vi "Set 430 Rate.vi"(8 "error in (no error)":errorcluster, 11 "VISA session":refnum<visa-resource-name>="GPIB0::22::INSTR") -> (0 "error out":errorcluster, 3 "VISA session out":refnum<visa-resource-name>="GPIB0::22::INSTR")   [LabVIEW 2021]
panel:
  in  "Slew Rate [T/min]":dbl
  in  "Input Cluster":T1 {"MaxLambdaCurrent [A]" format="%.2f"; "LambdaRates [A/min]" format="%.5e"; "MaxNormalCurrent [A]" format="%.2f"; "StabilitySetting [%]" format="%.2f"; "FieldCurrentRatio [T/A]" format="%.2f"; "SwitchWaitTime [s]" format="%.2f"; "SwitchHtrCurrent [mA]" format="%.2f"; "TrainRates [A/min]" format="%.5e"; "NormalRates [A/min]" format="%.5e"; "Breakpts [A]" format="%.5e"}
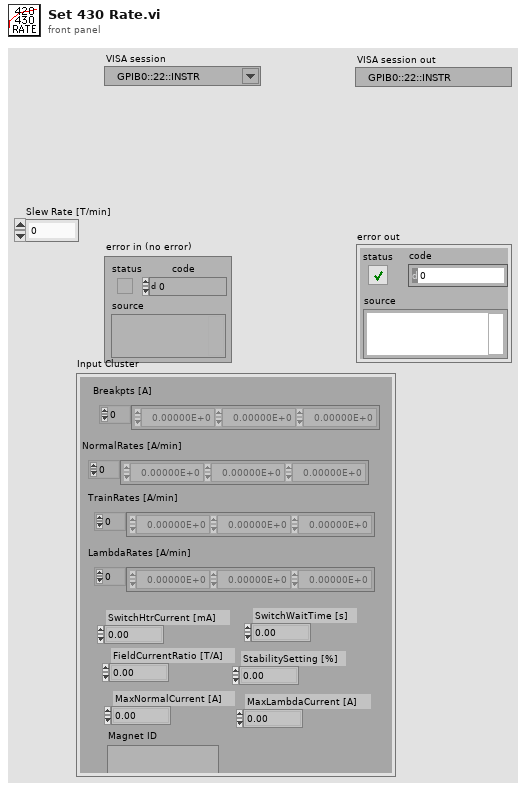
[diagram p1: front panel]
types:
  T1 = cluster{"Breakpts [A]":dbl[], "NormalRates [A/min]":dbl[], "TrainRates [A/min]":dbl[], "SwitchHtrCurrent [mA]":dbl, "SwitchWaitTime [s]":dbl, "FieldCurrentRatio [T/A]":dbl, "StabilitySetting [%]":dbl, "MaxNormalCurrent [A]":dbl, "Magnet ID":string, "LambdaRates [A/min]":dbl[], "MaxLambdaCurrent [A]":dbl}
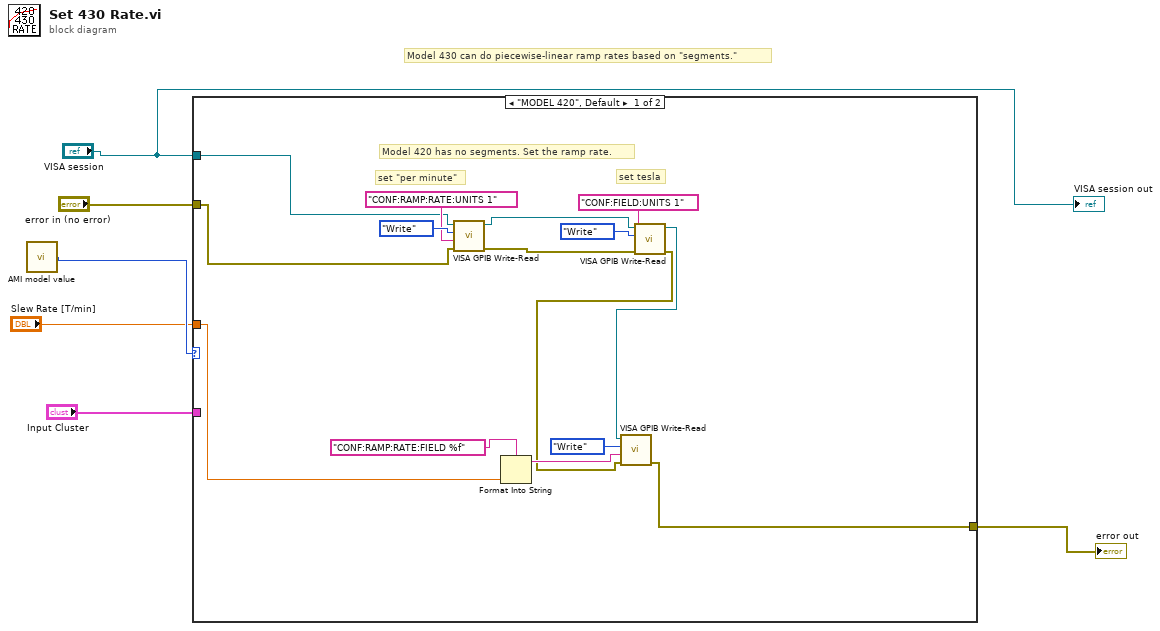
[diagram p0: block diagram]
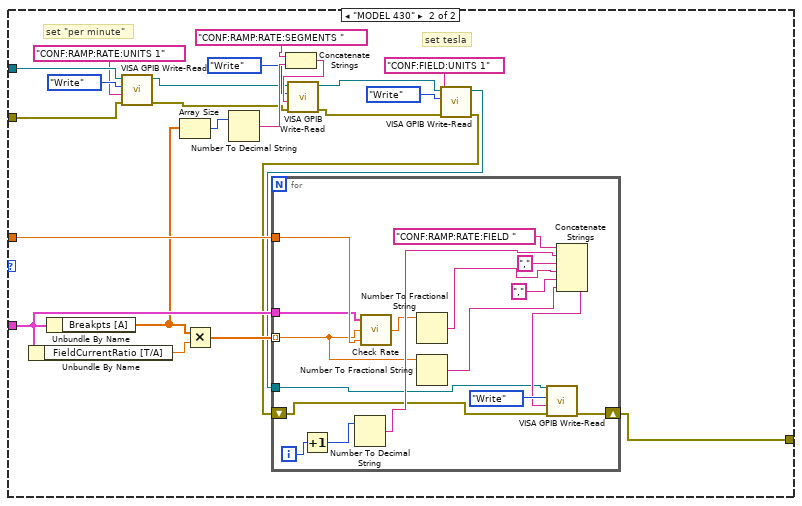
[diagram p2: hidden frame]
diagram:
  # "Model 430 can do piecewise-linear ramp rates based on \"segments.\""
  n1 = call "AMI model value.vi"() -> ("AMI Model 2"=w3:enum16{"MODEL 420", "MODEL 430"})  [unwired: 2 in]
  n2 = case shown="\"MODEL 420\", Default" w3 {
    tunnel: "VISA session" -> [w9 w42]
    tunnel: "error in (no error)" -> [w10 w41]
    tunnel: [w18 w24] -> w5
    tunnel: "Input Cluster" -> [_ w37]
    tunnel: "Slew Rate [T/min]" -> [w17 w38]
    frame "MODEL 420", Default {
      # "set tesla"
      # "set \"per minute\""
      # "Model 420 has no segments. Set the ramp rate."
      n3 = call "VISA GPIB Write-Read.vi"("error in (no error)"=w10, "Command"="CONF:RAMP:RATE:UNITS 1" ("Command String"), "Action"=enum16{"Write", "Read", "Write & Read"}."Write", "VISA resource name"=w9) -> ("error out"=w11:errorcluster, "dup VISA Session"=w12:refnum<visa-resource-name>)  [unwired: 4 in, 2 out]
      n4 = Format Into String(format string="CONF:RAMP:RATE:FIELD %f" ("Command String"), w17) -> (resulting string=w20:string)  [unwired: 2 in, 1 out]
      n5 = call "VISA GPIB Write-Read.vi"("error in (no error)"=w11, "Command"="CONF:FIELD:UNITS 1" ("Command String"), "Action"=enum16{"Write", "Read", "Write & Read"}."Write", "VISA resource name"=w12) -> ("error out"=w8:errorcluster, "dup VISA Session"=w7:refnum<visa-resource-name>)  [unwired: 4 in, 2 out]
      n6 = call "VISA GPIB Write-Read.vi"("error in (no error)"=w8, "Command"=w20, "Action"=enum16{"Write", "Read", "Write & Read"}."Write", "VISA resource name"=w7) -> ("error out"=w18:errorcluster)  [unwired: 4 in, 3 out]
    }
    frame "MODEL 430" {
      # "set tesla"
      # "set \"per minute\""
      n7 = Unbundle By Name(w37) -> ("FieldCurrentRatio [T/A]"=w44:dbl)
      n8 = Unbundle By Name(w37) -> ("Breakpts [A]"=w33:dbl[])
      n9 = call "VISA GPIB Write-Read.vi"("error in (no error)"=w41, "Command"="CONF:RAMP:RATE:UNITS 1" ("Command String"), "Action"=enum16{"Write", "Read", "Write & Read"}."Write", "VISA resource name"=w42) -> ("error out"=w29:errorcluster, "dup VISA Session"=w30:refnum<visa-resource-name>)  [unwired: 4 in, 2 out]
      n10 = Array Size(array=w33) -> (size(s)=w36:i32)
      n11 = Multiply(x=w33, y=w44) -> (x*y=w39:dbl[])
      n12 = Number To Decimal String(number=w36) -> (decimal integer string=w34:string)  [unwired: 1 in]
      n13 = Concatenate Strings("CONF:RAMP:RATE:SEGMENTS " ("Command String"), w34) -> (w32:string)
      n14 = call "VISA GPIB Write-Read.vi"("error in (no error)"=w29, "Command"=w32, "Action"=enum16{"Write", "Read", "Write & Read"}."Write", "VISA resource name"=w30) -> ("error out"=w25:errorcluster, "dup VISA Session"=w26:refnum<visa-resource-name>)  [unwired: 4 in, 2 out]
      n15 = call "VISA GPIB Write-Read.vi"("error in (no error)"=w25, "Command"="CONF:FIELD:UNITS 1" ("Command String"), "Action"=enum16{"Write", "Read", "Write & Read"}."Write", "VISA resource name"=w26) -> ("error out"=w23:errorcluster, "dup VISA Session"=w22:refnum<visa-resource-name>)  [unwired: 4 in, 2 out]
      n16 = for {
        tunnel: w39 -> [w51] mode=indexing
        tunnel: w38 -> [w61]
        tunnel: w37 -> [w60]
        shift-right: [w47] -> w24
        shift-left: w23 -> [w46]
        tunnel: w22 -> [w45]
        i -> [w59]
        n17 = Increment(x=w59) -> (x+1=w58:i32)
        n18 = Number To Decimal String(number=w58) -> (decimal integer string=w56:string)  [unwired: 1 in]
        n19 = call "Check Rate.vi"("Rate"=w61, "Field"=w51, "input cluster"=w60) -> ("Checked Rate"=w54:dbl)
        n20 = Number To Fractional String(number=w54) -> (F-format string=w53:string)  [unwired: 3 in]
        n21 = Number To Fractional String(number=w51) -> (F-format string=w50:string)  [unwired: 3 in]
        n22 = Concatenate Strings("CONF:RAMP:RATE:FIELD " ("Command String"), w56, "," ("Command String"), w53, "," ("Command String"), w50) -> (w48:string)
        n23 = call "VISA GPIB Write-Read.vi"("error in (no error)"=w46, "Command"=w48, "Action"=enum16{"Write", "Read", "Write & Read"}."Write", "VISA resource name"=w45) -> ("error out"=w47:errorcluster)  [unwired: 4 in, 3 out]
      }
    }
  }
  "error out" <- w5
  "VISA session out" <- "VISA session"
